vi "SMO.jsonRPC.methodName.vi"(8 "error in (no error)":errorcluster, 10 "myData":string, 11 "SMO.ByRefWithEvents":refnum<class "SMO.jsonRPC.lvclass">) -> (0 "error out":errorcluster, 2 "Data Out":string, 3 "SMO.ByRefWithEvents out":refnum<class "SMO.jsonRPC.lvclass">)   [LabVIEW 2013, in "SMO.jsonRPC.lvclass"]
doc: "---------------------------------------------------------------\nJKI State Machine Objects™\nhttp://jki.net/state-machine-objects/\nCopyright (C) 2005-2015, JKI <info@jki.net>\nALL RIGHTS RESERVEDJKI State Machine Objects (SMO) 1.0.0.5\nJKI - JKI\nCopyright (c) 2016, JKI"
uses:
  SMO.jsonRPC.lvclass
  SMO.jsonRPC.lvclass/SMO.jsonRPC.ctl
panel:
  # "For instructions on how to use the JKI State Machine Objects, examples and video tutorials, visit:\nhttp://jki.net/state-machine-objects/\n\nJKI State Machine Objects™\nhttp://jki.net/state-machine-objects/\nCopyright (C) 2005-2015, JKI <info@jki.net>\nALL RIGHTS RESERVED"
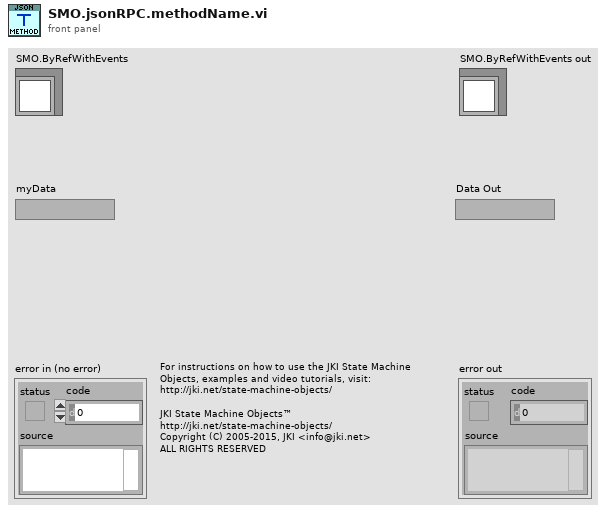
[diagram p1: front panel]
types:
  T1 = typedef "SMO.jsonRPC.lvclass/PrivateData--Ref.ctl" = refnum<data-value>
  T2 = typedef "SMO.jsonRPC.lvclass/PrivateData--Cluster.ctl" = cluster{"Public Events":T3, "Private Events":T4, "Data":string}
  T3 = typedef "SMO.jsonRPC.lvclass/PublicEvents--Cluster.ctl" = cluster{"Reply":refnum<user-event>}
  T4 = typedef "SMO.jsonRPC.lvclass/PrivateEvents--Cluster.ctl" = cluster{"Incoming Request":refnum<user-event>}
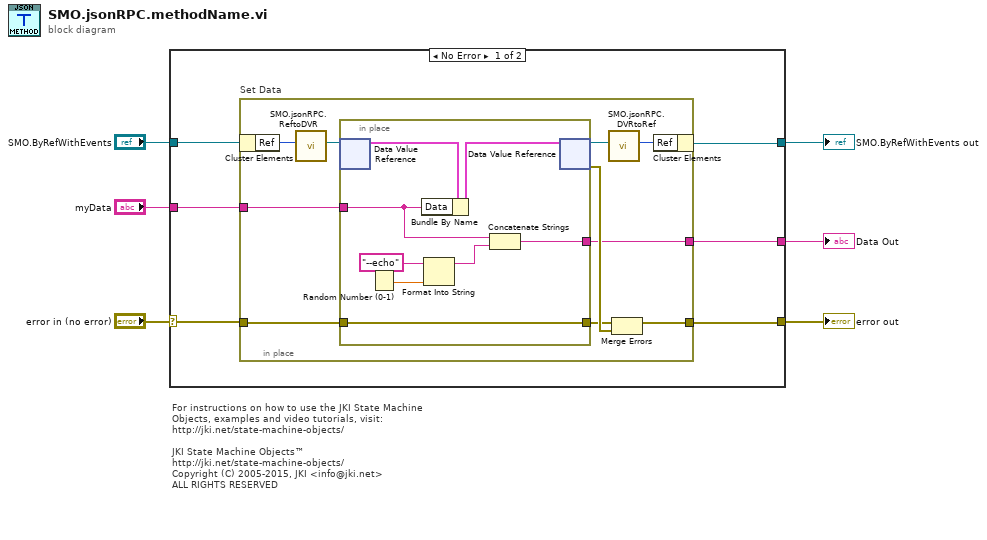
[diagram p0: block diagram]
diagram:
  # "For instructions on how to use the JKI State Machine Objects, examples and video tutorials, visit:\nhttp://jki.net/state-machine-objects/\n\nJKI State Machine Objects™\nhttp://jki.net/state-machine-objects/\nCopyright (C) 2005-2015, JKI <info@jki.net>\nALL RIGHTS RESERVED"
  n1 = case shown="No Error" "error in (no error)" {
    selector: "error in (no error)" -> [w10 w32]
    tunnel: "SMO.ByRefWithEvents" -> [w12 w33]
    tunnel: [w7 w32] -> w5
    tunnel: [w8 w33] -> w4
    tunnel: [w9 w31] -> w2
    tunnel: "myData" -> [w11 w31]
    frame No Error {
      n2 = in-place "Set Data" {
        in-place-border: w10 -> [w22]
        in-place-border: [w19] -> w7
        in-place-border: w11 -> [w14]
        in-place-border: [w13] -> w9
        n3 = in-place-cluster #1(w12) -> ("Ref"=w18:u32)
        n4 = call "SMO.jsonRPC.ReftoDVR.vi"("Ref"=w18) -> ("Ref"=w17:T1)  [unwired: 10 in]
        n5 = in-place {
          in-place-border: w22 -> [w30]
          in-place-border: [w30] -> w20
          in-place-border: w14 -> [w27]
          in-place-border: [w26] -> w13
          n6 = in-place-dvr #2(w17) -> (w28:T2)  [unwired: 1 out]
          n7 = Random Number (0-1)() -> (number: 0 to 1=w25:dbl)
          n8 = Bundle By Name(cluster=w28, "Data"=w27) -> (w29:T2)
          n9 = Format Into String(initial string="--echo", w25) -> (resulting string=w23:string)  [unwired: 2 in, 1 out]
          n10 = Concatenate Strings(w27, w23) -> (w26:string)
          n11 = in-place-dvr #2(w29) -> (w16:T1, w21:errorcluster)
        }
        n12 = call "SMO.jsonRPC.DVRtoRef.vi"("Ref"=w16) -> ("Ref"=w15:u32)  [unwired: 10 in]
        n13 = Merge Errors(w20, w21) -> (w19:errorcluster)
        n14 = in-place-cluster #1("Ref"=w15) -> (w8:refnum<class "SMO.jsonRPC.lvclass">)
      }
    }
    frame Error {
    }
  }
  "error out" <- w5
  "SMO.ByRefWithEvents out" <- w4
  "Data Out" <- w2
